vi "set_danger_accept_invalid_certs.vi"(8 "error in (no error)":errorcluster, 10 "danger_accept_invalid_certs":bool, 11 "ClientBuilder in":refnum<class "ClientBuilder.lvclass">) -> (0 "error out":errorcluster, 2 "success":bool, 3 "ClientBuilder out":refnum<class "ClientBuilder.lvclass">)   [LabVIEW 2020, in "reqwest.lvlib" / "ClientBuilder.lvclass"]
uses:
  ClientBuilder.lvclass
  ClientBuilder.lvclass/ClientBuilder.ctl
  lv_reqwest_64.dll
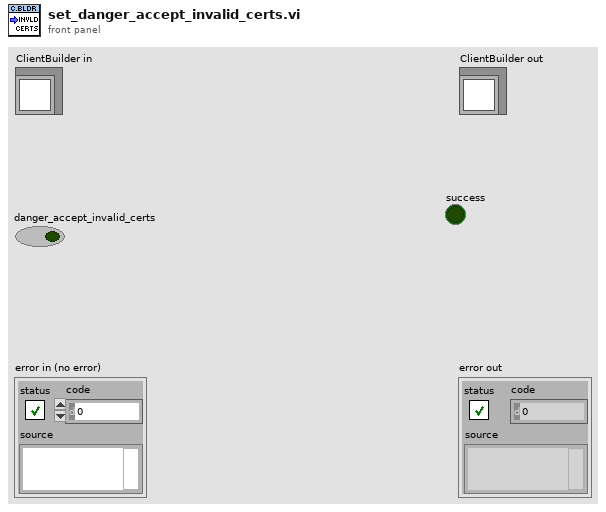
[diagram p1: front panel]
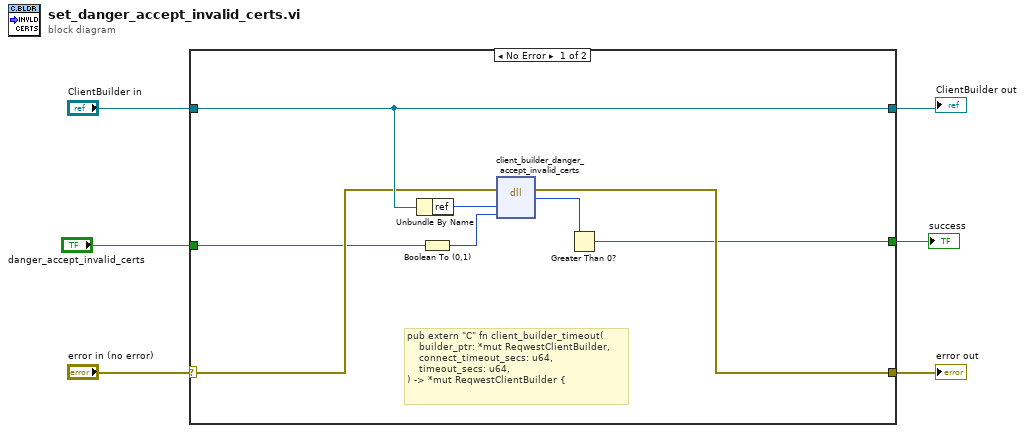
[diagram p0: block diagram]
diagram:
  n1 = case shown="No Error" "error in (no error)" {
    selector: "error in (no error)" -> [w11 w15]
    tunnel: "ClientBuilder in" -> [w12 w16]
    tunnel: [w14 w15] -> w3
    tunnel: [w12 w16] -> w4
    tunnel: "danger_accept_invalid_certs" -> [w8 _]
    tunnel: [w9 _] -> w1
    frame No Error {
      # "pub extern \"C\" fn client_builder_timeout(\n    builder_ptr: *mut ReqwestClientBuilder,\n    connect_timeout_secs: u64,\n    timeout_secs: u64,\n) -> *mut ReqwestClientBuilder {"
      n2 = Unbundle By Name(w12) -> ("ref"=w13:u64)
      n3 = Boolean To (0,1)(Boolean=w8) -> (0, 1=w7:i16)
      n4 = dll-call lib="C:/Projects/reqwest-rs-labview/lv_src/lv_reqwest_*.*" fn="client_builder_danger_accept_invalid_certs"(error in=w11, "client_builder_ref"=w13, "danger_accept_invalid_certs"=w7) -> (error out=w14:errorcluster, "success"=w10:u8)  [unwired: 4 in, 1 out]
      n5 = Greater Than 0?(x=w10) -> (x > 0?=w9:bool)
    }
    frame Error {
    }
  }
  "error out" <- w3
  "ClientBuilder out" <- w4
  "success" <- w1
